vi "DesiredString2DesiredBundle.vi"(0 "ParameterSet":string) -> (4 "DesiredParameters":T1, 8 "Controller?":bool)   [LabVIEW 2019]
uses:
  TypeDef/Command Cluster.ctl
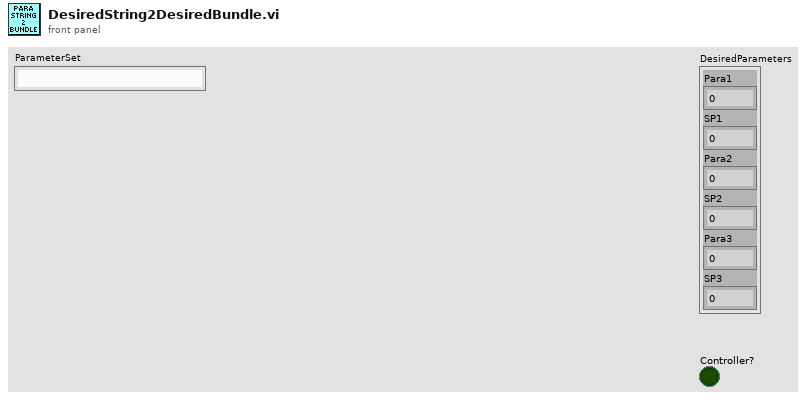
[diagram p1: front panel]
types:
  T1 = typedef "Command Cluster.ctl" = cluster{"Para1":i32, "SP1":dbl, "Para2":i32, "SP2":dbl, "Para3":i32, "SP3":dbl}
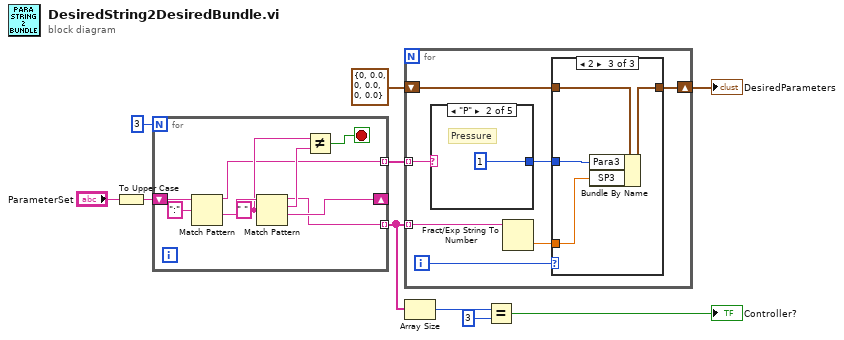
[diagram p0: block diagram]
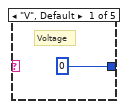
[diagram p2: hidden frame]
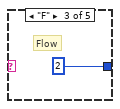
[diagram p3: hidden frame]
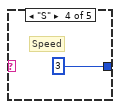
[diagram p4: hidden frame]
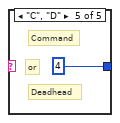
[diagram p5: hidden frame]
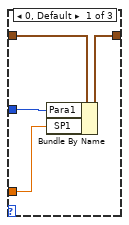
[diagram p6: hidden frame]
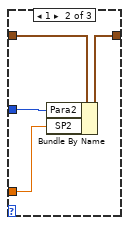
[diagram p7: hidden frame]
diagram:
  n1 = To Upper Case(1:"ParameterSet") -> (0:w6:string)
  n2 = for {
    N: 3 -> [_]
    shift-right: [w12] -> _
    shift-left: w6 -> [w19]
    tunnel: [w11] -> w4 mode=indexing
    tunnel: [w13] -> w7 mode=indexing
    stop <- w14 stop-if-true
    w16 = " " ("regular expression")
    n3 = Match Pattern(string=w19, regular expression=":") -> (before substring=w13:string, after substring=w17:string)  [unwired: 1 in, 2 out]
    n4 = Match Pattern(string=w17, regular expression=w16) -> (before substring=w11:string, match substring=w15:string, after substring=w12:string)  [unwired: 1 in, 1 out]
    n5 = Not Equal?(x=w16, y=w15) -> (x != y?=w14:bool)
  }
  n6 = for {
    tunnel: w4 -> [w25] mode=indexing
    tunnel: w7 -> [w23] mode=indexing
    shift-right: [w21] -> w9
    shift-left: T1 {"Para1"=0, "SP1"=0.0, "Para2"=0, "SP2"=0.0, "Para3"=0, "SP3"=0.0} ("CMDCluster In") -> [w22]
    i -> [w26]
    n7 = case shown="\"P\"" w23 {
      tunnel: [0 ("Para1") 1 ("Para1") 2 ("Para1") 3 ("Para1") 4 ("Para1")] -> w20
      frame "V", Default {
        # "Voltage"
      }
      frame "P" {
        # "Pressure"
      }
      frame "F" {
        # "Flow"
      }
      frame "S" {
        # "Speed"
      }
      frame "C", "D" {
        # "or"
        # "Deadhead"
        # "Command"
      }
    }
    n8 = Fract/Exp String To Number(string=w25) -> (number=w24:dbl)  [unwired: 3 in, 1 out]
    n9 = case shown="2" w26 {
      tunnel: w24 -> [w32 w36 w40]
      tunnel: w22 -> [w35 w39 w43]
      tunnel: [w34 w38 w42] -> w21
      tunnel: w20 -> [w33 w37 w41]
      frame 0, Default {
        n10 = Bundle By Name(cluster=w35, "Para1"=w33, "SP1"=w32) -> (w34:T1)
      }
      frame 1 {
        n11 = Bundle By Name(cluster=w39, "Para2"=w37, "SP2"=w36) -> (w38:T1)
      }
      frame 2 {
        n12 = Bundle By Name(cluster=w43, "Para3"=w41, "SP3"=w40) -> (w42:T1)
      }
    }
  }
  "DesiredParameters" <- w9
  n13 = Array Size(array=w4) -> (size(s)=w3:i32)
  n14 = Equal?(x=w3, y=3) -> (x = y?=→"Controller?":bool)
